vi "Initialize and Run FPGA VI.vi"(8 "error in (no error)":errorcluster, 10 "Timeout Period (ticks)":u64, 11 "Control Period (ticks)":u32) -> (0 "error out":errorcluster, 3 "FPGA VI Reference Out":T1)   [LabVIEW 2014]
uses:
  <vilib>/rvi/interface/nirviOpenFPGA/nirviOpenFPGA.xnode
  <vilib>/rvi/interface/nirviReadWriteControl/nirviReadWriteControl.xnode
  <vilib>/rvi/interface/nirviMethod/nirviMethod.xnode
  <vilib>/FPGAPlugInAG/Dynamic/niLvFpga_Reset_Dynamic.vi
  <vilib>/FPGAPlugInAG/Dynamic/niLvFpga_Run_Dynamic.vi
  NiFpgaLv.dll
  <vilib>/Utility/error.llb/Error Cluster From Error Code.vi
  <vilib>/rvi/interface/Simulation/niFpgaSimulationCallBeginRW.vi
  <vilib>/rvi/errors/niLvFpgaAdjustHostInterfaceError.vi
  FPGA Bitfiles/FPGAControlonCom_FPGATarget_FPGAMain_278E7659.lvbitx
  FPGA Main.vi
  <vilib>/FPGAPlugInAG/cRIO-9074/niLvFpga_Open_cRIO-9074.vi
  <vilib>/rvi/interface/common/dynamic/niFpgaDynamicAddResources.vi
  controls/FPGA VI Reference.ctl
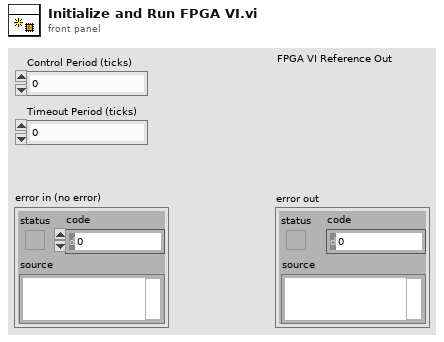
[diagram p1: front panel]
types:
  T1 = typedef "FPGA VI Reference.ctl" = refnum<k20>
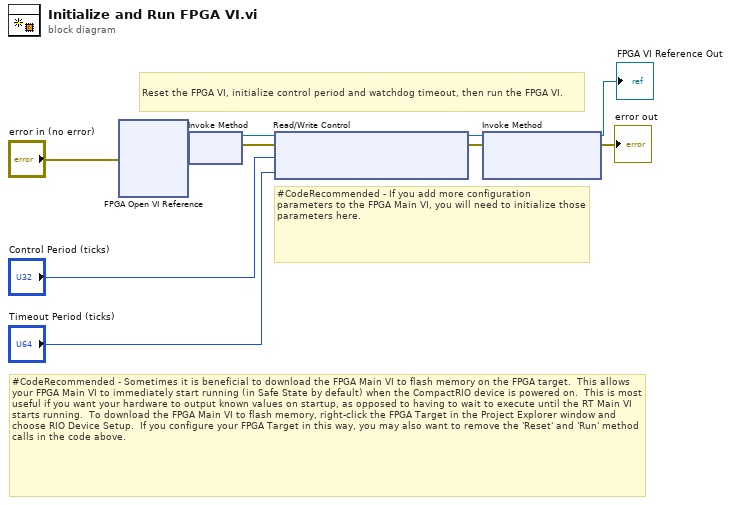
[diagram p0: block diagram]
diagram:
  # "#CodeRecommended - Sometimes it is beneficial to download the FPGA Main VI to flash memory on the FPGA target.  This allows your FPGA Main VI to immediately start running (in Safe State by default) when the CompactRIO device is powered on.  This is most useful if you want your hardware to output known values on startup, as opposed to having to wait to execute until the RT Main VI starts running.  To download the FPGA Main VI to flash memory, right-click the FPGA Target in the Project Explorer window and choose RIO Device Setup.  If you configure your FPGA Target in this way, you may also want to remove the 'Reset' and 'Run' method calls in the code above."
  # "Reset the FPGA VI, initialize control period and watchdog timeout, then run the FPGA VI."
  # "#CodeRecommended - If you add more configuration parameters to the FPGA Main VI, you will need to initialize those parameters here."
  n1 = xnode "FPGA Open VI Reference"("error in"="error in (no error)") -> ("FPGA VI Reference Out"=w1:refnum<k20>, "error out"=w2:errorcluster)  [unwired: 1 in]
  n2 = xnode "Invoke Method"("FPGA VI Reference In"=w1, "error in"=w2) -> ("FPGA VI Reference Out"=w3:refnum<k20>, "error out"=w4:errorcluster)
  n3 = xnode "Read/Write Control"("FPGA VI Reference In"=w3, "error in"=w4, "Control Period (ticks)"="Control Period (ticks)", "Watchdog Timeout Period (ticks)"="Timeout Period (ticks)") -> ("FPGA VI Reference Out"=w7:refnum<k20>, "error out"=w8:errorcluster)
  n4 = xnode "Invoke Method"("FPGA VI Reference In"=w7, "error in"=w8) -> ("FPGA VI Reference Out"=→"FPGA VI Reference Out":refnum<k20>, "error out"=→"error out":errorcluster)  [unwired: 1 in]
